vi "New Acquire.vi"() -> ()   [LabVIEW 2019]
uses:
  <vilib>/vision/NI_Vision_Development_Module.lvlib
panel:
  in  "Tab Control":T1(tab)
  out "Counts per Laser Shot :":dbl format="%#.1g"
  in  "Image Size (pixels) :":dbl=400.0
  in  "?":bool
  in  "Acquiring :":bool
  in  "Save?":bool
  in  "Mask Width (pixels) :":dbl
  in  "Mask Centre :":bool
  in  "Threshold Level (%) :":dbl
  in  "Image Centre (x,y) : 2":dbl=250.0
  in  "Image Centre (x,y) :":dbl=301.0
  in  "Symmetrise L/R :":bool
  in  "Symmetrise U/D :":bool
  in  "Centroiding :":bool
  out "Test View":dbl[][](graph)
  out "Integrated Signal Graph":dbl[](graph)
  out "Live Camera View":dbl[][](graph)
  out "PECD = LCP - RCP":dbl[][](graph)
  out "RCP":dbl[][](graph)
  out "LCP":dbl[][](graph)
  out "Elipticity :":dbl format="%#.2g"
  in  "RCP Position :":dbl=85.7
  in  "?":refnum<k7>(container)
  in  "?":refnum<k7>(container)
  out "of":dbl
  out "Scan :":dbl
  out "Progress :":u8(slide) scale=0.0..100.0
  out "of":dbl
  out "Shot :":dbl
  in  "Molecule :":string
  in  "OK Button 2":bool
  in  "No. of CPL Cycles :":dbl=1.0
  in  "Shots per Cycle :":dbl=100.0
  in  "HWP Zero Position :":dbl=3.9
  out "?":cluster{dbl[], dbl[]}(graph)
  out "PEELD = LEP - REP":dbl[][](graph)
  out "REP Image":dbl[][](graph)
  out "LEP Image":dbl[][](graph)
  out "?":dbl[](graph)
  in  "HWP Step Size :":dbl=2.5
  in  "LCP Position :":dbl=175.7
  in  "No. of Scans :":dbl=10.0
  out "Shot :":dbl
  out "of":dbl
  out "Elipticity : 2":dbl format="%#.2g"
  in  "RCP Position : 2":dbl=85.7
  in  "?":refnum<k7>(container)
  in  "?":refnum<k7>(container)
  out "of  3":dbl
  out "Scan : 2":dbl
  out "Progress : 2":u8(slide) scale=0.0..100.0
  out "of  3":dbl
  out "Shot : 3":dbl
  in  "Molecule : 2":string
  in  "OK Button 3":bool
  in  "No. of CPL Cycles : 2":dbl=1.0
  in  "Shots per Cycle : 2":dbl=100.0
  in  "HWP Zero Position : 2":dbl=3.9
  out "?":cluster{dbl[], dbl[]}(graph)
  out "PEELD = LEP - REP 2":dbl[][](graph)
  out "REP Image 2":dbl[][](graph)
  out "LEP Image 2":dbl[][](graph)
  out "?":dbl[](graph)
  in  "HWP Step Size : 2":dbl=2.5
  in  "LCP Position : 2":dbl=175.7
  in  "No. of Scans : 2":dbl=10.0
  out "Shot : 2":dbl
  out "of 2":dbl
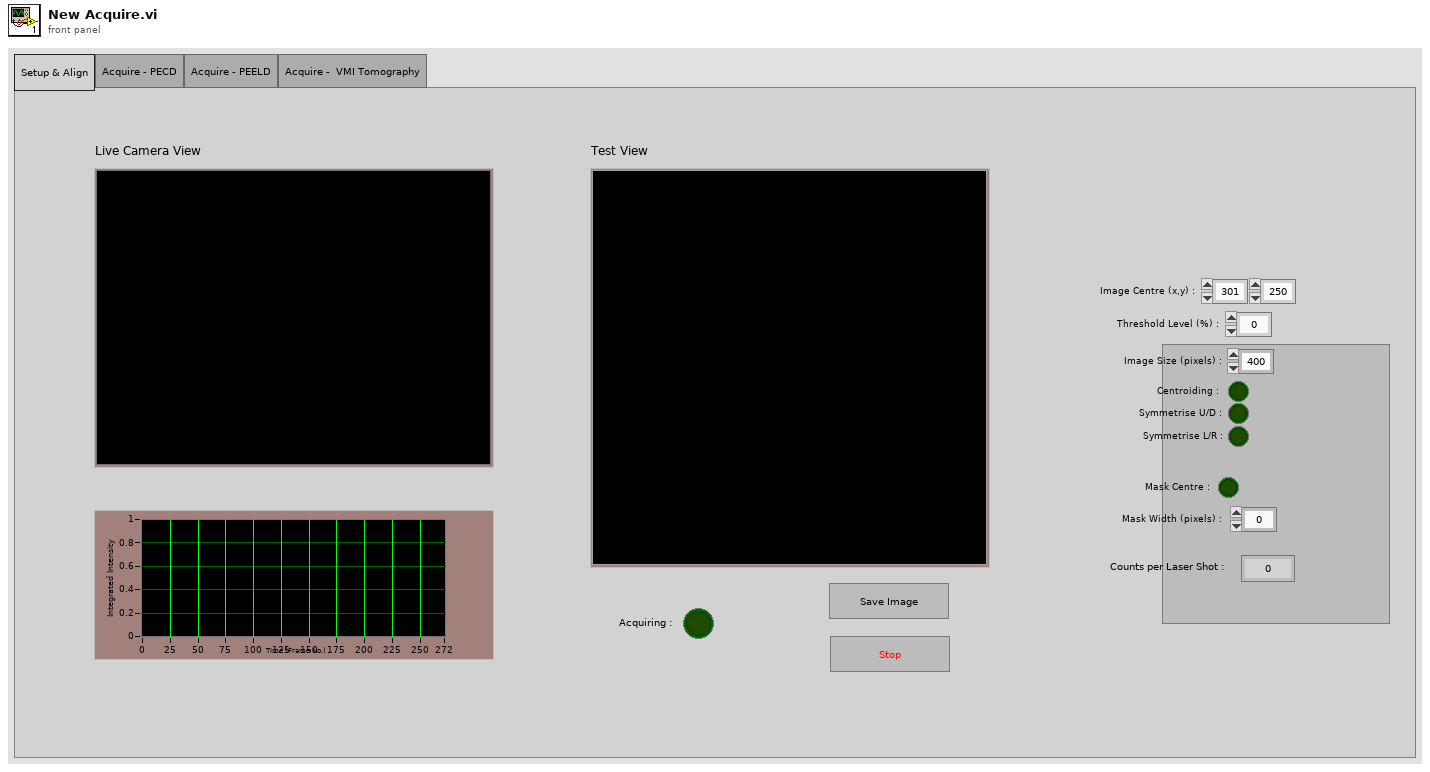
[diagram p1: front panel]
types:
  T1 = enum32{"Setup & Align", "Acquire - PECD", "Acquire - PEELD", "Acquire -  VMI Tomography"}
  T2 = typedef "Image Type" = u32
  T3 = typedef "IMAQ Image.ctl" = refnum<image>
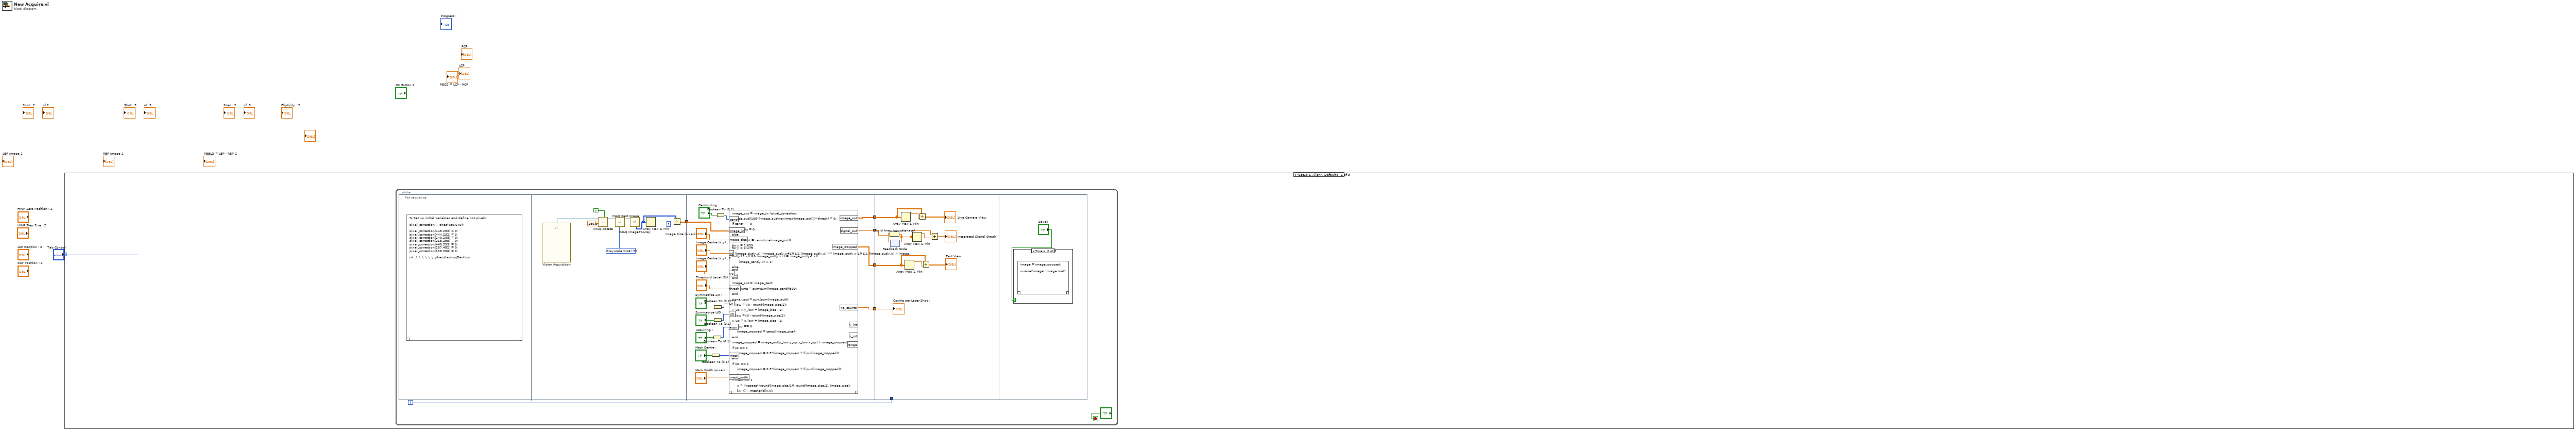
[diagram p0: block diagram]
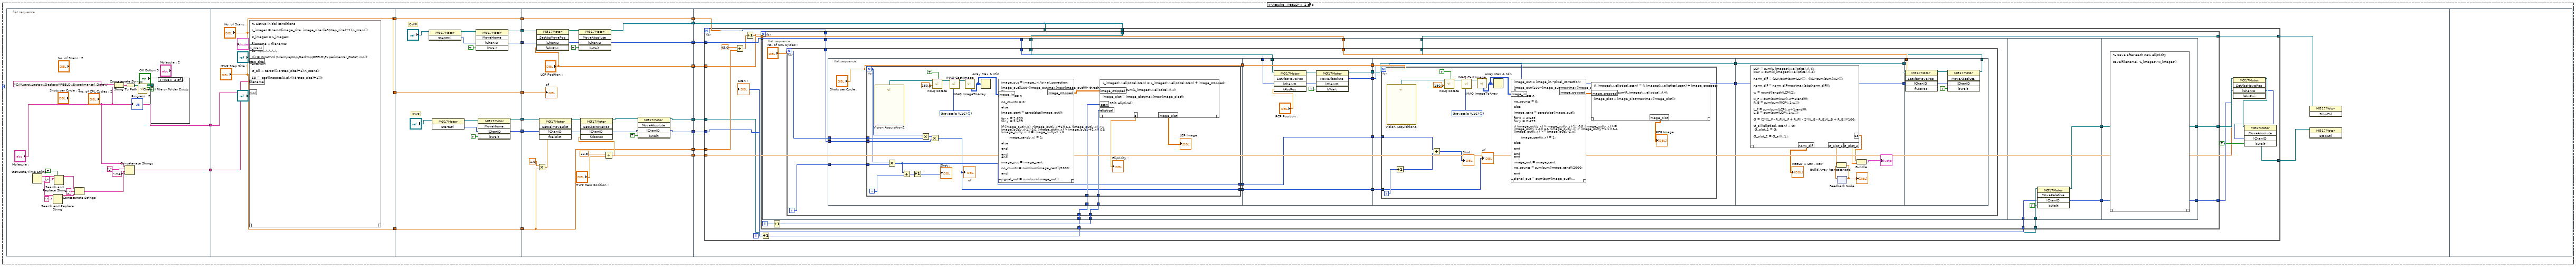
[diagram p3: hidden frame]
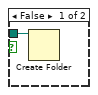
[diagram p4: hidden frame]
diagram:
  n1 = case shown="\"Setup & Align\", Default" "Tab Control" {
    frame "Setup & Align", Default {
      n2 = while {
        i -> [w4]
        stop <- "?" stop-if-true
        n3 = flat-sequence {
          tunnel: [w9] -> w8
          tunnel: w8 -> [w37]
          tunnel: [w36] -> w7
          tunnel: [w35] -> w5
          tunnel: [w31] -> w3
          tunnel: [w18] -> w2
          tunnel: w7 -> [w44]
          tunnel: w5 -> [w40]
          tunnel: w4 -> [_]
          tunnel: w3 -> [w41]
          tunnel: w2 -> [w38]
          frame #0 {
            n4 = script code="% Set up initial variables and define hot pixels\n\npixel_correction = ones(480,640);\n\npixel_correction(445,233) = 0;\npixel_correction(444,232) = 0\npixel_correction(240,208) = 0;\npixel_correction(268,295) = 0;\npixel_correction(440,333) = 0;\npixel_correction(257,482) = 0;\npixel_correction(128,286) = 0;\n\ncd ..\\..\\..\\..\\..\\..\\..\\Users\\Laptop\\Desktop"() -> ()  [unwired: 1 in, 1 out]
          }
          frame #1 {
            w17 = T2 7 items=["Grayscale (U8)", "Grayscale (I16)", "Grayscale (SGL)", "Complex (CSG)", "RGB (U32)", "HSL (U32)", "RGB (U64)", "Grayscale (U16)"] ("Image Type")
            n5 = call "Vision Acquisition"() -> ("Image Out"=w11:T3)  [unwired: 26 in, 1 out]
            n6 = call "IMAQ Rotate"("Maintain Size"=TRUE, "Angle (degrees)"=sgl 180.0, "Image Src"=w11) -> ("Image Dst Out"=w14:T3)  [unwired: 7 in, 1 out]
            n7 = call "IMAQ Cast Image"("Image Type"=w17, "Image Src"=w14) -> ("Image Dst Out"=w16:T3)  [unwired: 8 in, 1 out]
            n8 = call "IMAQ ImageToArray"("Image"=w16) -> ("Image Pixels (U16)"=w15:u16[][])  [unwired: 3 in, 4 out]
            n9 = Array Max & Min(array=w15) -> ()  [unwired: 4 out]
            n10 = Divide(x=w15, y=1) -> (x/y=w9:dbl[][])
          }
          frame #2 {
            n11 = Boolean To (0,1)(Boolean="Mask Centre :") -> (0, 1=w22:i16)
            n12 = Boolean To (0,1)(Boolean="Acquiring :") -> (0, 1=w25:i16)
            n13 = Boolean To (0,1)(Boolean="Symmetrise U/D :") -> (0, 1=w26:i16)
            n14 = Boolean To (0,1)(Boolean="Symmetrise L/R :") -> (0, 1=w29:i16)
            n15 = Boolean To (0,1)(Boolean="Centroiding :") -> (0, 1=w19:i16)
            n16 = script code="image_out = image_in.*pixel_correction;\n\nimage_out((100*(image_out/max(max(image_out))))<thresh) = 0;\n\nif centr == 0\n\nno_counts = 0;\n\nelse\n\nimage_cent = zeros(size(image_out));\n\nfor x = 2:639\nfor y = 2:479\n\nif (image_out(y,x) >image_out(y,x+1)) && (image_out(y,x) >= image_out(y,x-1)) && (image_out(y,x) > image_out(y+1,x)) && (image_out(y,x) >= image_out(y-1,x))\n\n       image_cent(y,x) = 1;\n\nelse\nend\n\nend\nend\n\nimage_out = image_cent;\n\nno_counts = sum(sum(image_cent))/500;\n\nend\n\nsignal_out = sum(sum(image_out));\n\ny_low = y0 - round(image_size/2);\n\ny_up = y_low + image_size - 1;\n\nx_low =x0 - round(image_size/2);\n\nx_up = x_low + image_size - 1;\n\nif acqu == 0\n\n     image_cropped = zeros(image_size);\n\nend\n\nimage_cropped = image_out(y_low:y_up,x_low:x_up) + image_cropped;\n\nif LR == 1\n\n     image_cropped = 0.5*(image_cropped + fliplr(image_cropped));\n\nend\n\nif UD == 1\n\n     image_cropped = 0.5*(image_cropped + flipud(image_cropped));\n\nend\n\nif mask == 1\n\n     x = linspace(-(round(image_size/2)), round(image_size/2), image_size);\n\n     [X, Y] = meshgrid(x,x);\n\n     R = sqrt(X.^2 + Y.^2);\n\n     mask_ = ones(size(R));\n\n     mask_(R<mask_width) = 0;\n\n     image_cropped = image_cropped.*mask_;\n\nend\n\nrange = 1:image_size;\n\ny_int = sum(image_cropped,1);\ny_int = y_int/max(y_int);\n\nx_int = sum(image_cropped,2);\nx_int = x_int/max(x_int);"("image_in"=w37, "image_size"="Image Size (pixels) :", "x0"="Image Centre (x,y) :", "y0"="Image Centre (x,y) : 2", "thresh"="Threshold Level (%) :", "LR"=w29, "UD"=w26, "acqu"=w25, "mask"=w22, "mask_width"="Mask Width (pixels) :", "centr"=w19) -> ("image_out"=w36:dbl[][], "signal_out"=w35:dbl, "image_cropped"=w31:dbl[][], "no_counts"=w18:dbl)  [unwired: 1 in, 4 out]
          }
          frame #3 {
            n17 = feedback #1() -> (w39:dbl[])  [unwired: 1 in]
            n18 = Build Array (concatenate)(w39, w40) -> (w48:dbl[])
            n19 = feedback-in #1(w48) -> ()
            n20 = Array Max & Min(array=w44) -> (max value=w45:dbl)  [unwired: 3 out]
            n21 = Array Max & Min(array=w41) -> (max value=w43:dbl)  [unwired: 3 out]
            n22 = Array Max & Min(array=w48) -> (max value=w47:dbl)  [unwired: 3 out]
            n23 = Divide(x=w44, y=w45) -> (x/y=→"Live Camera View":dbl[][])
            n24 = Divide(x=w41, y=w43) -> (x/y=→"Test View":dbl[][])
            n25 = Divide(x=w48, y=w47) -> (x/y=→"Integrated Signal Graph":dbl[])
            "Counts per Laser Shot :" <- w38
          }
          frame #4 {
            n26 = case shown="True" "Save?" {
              frame False {
              }
              frame True {
                n27 = script code="image = image_cropped;\n\nuisave('image','image.mat')"() -> ()  [unwired: 1 in, 1 out]
              }
            }
          }
        }
      }
    }
    frame "Acquire - PEELD" {
      n28 = flat-sequence {
        tunnel: [w72] -> w56
        tunnel: ["Molecule :"] -> w55
        tunnel: ["No. of Scans :"] -> w59
        tunnel: ["HWP Step Size :"] -> w57
        tunnel: w56 -> [w92]
        tunnel: w55 -> [w91]
        tunnel: ["No. of Scans :"] -> w53
        tunnel: [w100] -> w70
        tunnel: [w99] -> w69
        tunnel: [w98] -> w68
        tunnel: [w97] -> w67
        tunnel: [w96] -> w60
        tunnel: w59 -> [w96]
        tunnel: [w95] -> w58
        tunnel: w57 -> [w95]
        tunnel: w53 -> [w94]
        tunnel: [w94] -> w52
        tunnel: w70 -> [w133]
        tunnel: w69 -> [w132]
        tunnel: w68 -> [w131]
        tunnel: w67 -> [w130]
        tunnel: [w116] -> w66
        tunnel: [w122] -> w65
        tunnel: [w121] -> w64
        tunnel: ["LCP Position :"] -> w63
        tunnel: [w110] -> w62
        tunnel: [w119] -> w61
        tunnel: w60 -> [w119]
        tunnel: w58 -> [w110]
        tunnel: [w115] -> w54
        tunnel: w52 -> [w113]
        tunnel: [w112] -> w51
        tunnel: w66 -> [w143]
        tunnel: w65 -> [w139]
        tunnel: w64 -> [w141]
        tunnel: w63 -> [w140]
        tunnel: w62 -> [w136]
        tunnel: w61 -> [w135]
        tunnel: w54 -> [w142]
        tunnel: w51 -> [w134]
        frame #0 {
          n29 = Get Date/Time String() -> (date string=w83:string, time string=w80:string)  [unwired: 3 in]
          n30 = Search and Replace String(input string=w80, search string=":") -> (result string=w77:string)  [unwired: 6 in, 3 out]
          n31 = Search and Replace String(replace all?=TRUE ("replace all? (F)"), input string=w83, search string="/") -> (result string=w78:string)  [unwired: 5 in, 3 out]
          n32 = Concatenate Strings(w78, "_" ("string"), w77) -> (w74:string)
          n33 = Concatenate Strings("C:\\Users\\Laptop\\Desktop\\PEELD\\Experimental_Data\\", "Molecule :") -> (w84:string)
          n34 = Concatenate Strings("Molecule :", "_" ("string"), w74, ".mat" ("string")) -> (w72:string)
          n35 = String To Path(string=w84) -> (path=w87:path)
          n36 = call <vilib>:"Check if File or Folder Exists.vi"("path"=w87) -> ("file or folder exists?"=w86:bool, "dup path"=w85:path)  [unwired: 8 in, 1 out]
          n37 = case shown="True" w86 {
            tunnel: w85 -> [w89 _]
            frame False {
              n38 = Create Folder(path (use dialog)=w89) -> ()  [unwired: 2 in, 3 out]
            }
            frame True {
            }
          }
        }
        frame #1 {
          n39 = script code="% Set up initial conditions\n\nL_images = zeros([image_size, image_size,((45/step_size)+1),n_scans]);\n\nR_images = L_images;\n\nfilename = filename;\n\ncd  ..\\..\\..\\..\\..\\..\\\n\ndir = strcat('cd \\Users\\Laptop\\Desktop\\PEELD\\Experimental_Data\\',mol);\n\neval(dir)\n\nG_all = zeros(((45/step_size)+1),n_scans);\n\nS3 = -cos(linspace(0,pi,((45/step_size)+1)));"("n_scans"="No. of Scans :", "step_size"="HWP Step Size :", "filename"=w92, "mol"=w91) -> ()  [unwired: 1 in, 1 out]
        }
        frame #2 {
          # "HWP"
          # "QWP"
          n40 = invoke class="MG17Motor" method="StartCtrl"(reference="?") -> (reference out=w106:refnum<k7>, "StartCtrl"=w105:i32)  [unwired: 2 in, 1 out]
          n41 = invoke class="MG17Motor" method="StartCtrl"(reference="?") -> (reference out=w103:refnum<k7>, "StartCtrl"=w102:i32)  [unwired: 2 in, 1 out]
          n42 = invoke class="MG17Motor" method="MoveHome"(reference=w106, "lChanID"=w105, "bWait"=TRUE) -> (reference out=w100:refnum<k7>, "lChanID"=w98:i32)  [unwired: 2 in, 3 out]
          n43 = invoke class="MG17Motor" method="MoveHome"(reference=w103, "lChanID"=w102, "bWait"=TRUE) -> (reference out=w99:refnum<k7>, "lChanID"=w97:i32)  [unwired: 2 in, 3 out]
        }
        frame #3 {
          n44 = invoke class="MG17Motor" method="SetAbsMovePos"(reference=w133, "lChanID"=w131, "fAbsPos"="LCP Position :") -> (reference out=w129:refnum<k7>, "lChanID"=w128:i32)  [unwired: 2 in, 3 out]
          n45 = Multiply(x=-1.0, y=w110) -> (x*y=w111:dbl)
          n46 = invoke class="MG17Motor" method="SetRelMoveDist"(reference=w132, "lChanID"=w130, "fRelDist"=w111) -> (reference out=w126:refnum<k7>, "lChanID"=w125:i32)  [unwired: 2 in, 3 out]
          n47 = invoke class="MG17Motor" method="MoveAbsolute"(reference=w129, "lChanID"=w128, "bWait"=TRUE) -> (reference out=w122:refnum<k7>, "lChanID"=w121:i32)  [unwired: 2 in, 3 out]
          n48 = Add(x=22.5, y="HWP Zero Position :") -> (x+y=w112:dbl)
          n49 = invoke class="MG17Motor" method="SetAbsMovePos"(reference=w126, "lChanID"=w125, "fAbsPos"=w112) -> (reference out=w118:refnum<k7>, "lChanID"=w117:i32)  [unwired: 2 in, 3 out]
          n50 = invoke class="MG17Motor" method="MoveAbsolute"(reference=w118, "lChanID"=w117, "bWait"=TRUE) -> (reference out=w116:refnum<k7>, "lChanID"=w115:i32)  [unwired: 2 in, 3 out]
          "of" <- w113
        }
        frame #4 {
          n51 = for {
            N: w135 -> [w155]
            tunnel: w143 -> [w146]
            tunnel: w142 -> [w147]
            tunnel: w139 -> [_]
            tunnel: w141 -> [w162]
            tunnel: w140 -> [w161]
            tunnel: w139 -> [w163]
            tunnel: [w160] -> w138
            tunnel: [w159] -> w137
            tunnel: w136 -> [w157]
            tunnel: w134 -> [w148]
            i -> [w156]
            n52 = Divide(x=45.0, y=w157) -> (x/y=w144:dbl)
            n53 = Increment(x=w144) -> (x+1=w145:dbl)
            n54 = Increment(x=w156) -> (x+1=w154:i32)
            "Scan :" <- w154
            n55 = for {
              N: w145 -> [_]
              tunnel: w163 -> [w177]
              tunnel: w162 -> [w176]
              tunnel: w161 -> [w175]
              tunnel: w146 -> [w174]
              tunnel: w147 -> [w173]
              tunnel: [w172] -> w151
              tunnel: [w171] -> w150
              tunnel: [w170] -> w160
              tunnel: w154 -> [w167]
              tunnel: w155 -> [w164]
              i -> [w169]
              n56 = flat-sequence {
                tunnel: w177 -> [w184]
                tunnel: w176 -> [w183]
                tunnel: w175 -> [w182]
                tunnel: [w181] -> w170
                tunnel: w168 -> [w180]
                tunnel: w167 -> [w179]
                tunnel: w164 -> [w178]
                tunnel: w174 -> [w287]
                tunnel: w173 -> [w286]
                tunnel: [w285] -> w166
                tunnel: [w284] -> w165
                tunnel: [w288] -> w171
                tunnel: [w289] -> w172
                tunnel: w166 -> [w289]
                tunnel: w165 -> [w288]
                frame #0 {
                  n57 = for {
                    N: "No. of CPL Cycles :" -> [w191]
                    tunnel: w184 -> [w204]
                    tunnel: w183 -> [w203]
                    tunnel: w182 -> [w200]
                    tunnel: [w199] -> w181
                    tunnel: w180 -> [w198]
                    tunnel: w179 -> [w197]
                    tunnel: w178 -> [w190]
                    i -> [w192]
                    n58 = flat-sequence {
                      tunnel: ["Shots per Cycle :"] -> w206
                      tunnel: w198 -> [w213]
                      tunnel: w197 -> [w212]
                      tunnel: w192 -> [w211]
                      tunnel: w191 -> [w210]
                      tunnel: w190 -> [w209]
                      tunnel: [w208] -> w189
                      tunnel: [w207] -> w187
                      tunnel: w206 -> [w247]
                      tunnel: [w247] -> w205
                      tunnel: w204 -> [w243]
                      tunnel: w203 -> [w242]
                      tunnel: [w240] -> w202
                      tunnel: [w239] -> w201
                      tunnel: w189 -> [w238]
                      tunnel: [w238] -> w188
                      tunnel: w187 -> [w237]
                      tunnel: [w237] -> w186
                      tunnel: w205 -> [w252]
                      tunnel: [w251] -> w196
                      tunnel: w202 -> [w251]
                      tunnel: w201 -> [w250]
                      tunnel: [w250] -> w194
                      tunnel: w188 -> [w249]
                      tunnel: w186 -> [w248]
                      tunnel: w196 -> [w275]
                      tunnel: [w275] -> w195
                      tunnel: w194 -> [w274]
                      tunnel: [w274] -> w193
                      tunnel: w195 -> [w279]
                      tunnel: w193 -> [w278]
                      tunnel: w200 -> [w277]
                      tunnel: [w276] -> w199
                      frame #0 {
                        n59 = for {
                          N: "Shots per Cycle :" -> [w218]
                          tunnel: w213 -> [w228]
                          tunnel: w212 -> [w227]
                          tunnel: w211 -> [w225]
                          tunnel: w210 -> [w221]
                          tunnel: w209 -> [w219]
                          tunnel: [w217] -> w208
                          tunnel: [w216] -> w207
                          i -> [w224]
                          w236 = T2 7 items=["Grayscale (U8)", "Grayscale (I16)", "Grayscale (SGL)", "Complex (CSG)", "RGB (U32)", "HSL (U32)", "RGB (U64)", "Grayscale (U16)"] ("Image Type")
                          n60 = call "Vision Acquisition2"() -> ("Image Out"=w231:T3)  [unwired: 26 in, 1 out]
                          n61 = Multiply(x=w218, y=w225) -> (x*y=w217:i32)
                          n62 = Add(x=w217, y=w224) -> (x+y=w223:i32)
                          n63 = Increment(x=w223) -> (x+1=→"Shot :":i32)
                          n64 = Multiply(x=w218, y=w221) -> (x*y=w220:i32)
                          n65 = Multiply(x=w220, y=w219) -> (x*y=w216:i32)
                          "of" <- w216
                          n66 = call "IMAQ Rotate"("Maintain Size"=TRUE, "Angle (degrees)"=sgl 180.0, "Image Src"=w231) -> ("Image Dst Out"=w234:T3)  [unwired: 7 in, 1 out]
                          n67 = call "IMAQ Cast Image"("Image Type"=w236, "Image Src"=w234) -> ("Image Dst Out"=w235:T3)  [unwired: 8 in, 1 out]
                          n68 = call "IMAQ ImageToArray"("Image"=w235) -> ("Image Pixels (U16)"=w230:u16[][])  [unwired: 3 in, 4 out]
                          n69 = Array Max & Min(array=w230) -> ()  [unwired: 4 out]
                          n70 = script code="image_out = image_in.*pixel_correction;\n\nimage_out((100*(image_out/max(max(image_out))))<thresh) = 0;\n\nif centr == 0\n\nno_counts = 0;\n\nelse\n\nimage_cent = zeros(size(image_out));\n\nfor x = 2:639\nfor y = 2:479\n\nif (image_out(y,x) >image_out(y,x+1)) && (image_out(y,x) >= image_out(y,x-1)) && (image_out(y,x) > image_out(y+1,x)) && (image_out(y,x) >= image_out(y-1,x))\n\n       image_cent(y,x) = 1;\n\nelse\n\nend\n\nend\nend\n\nimage_out = image_cent;\n\nno_counts = sum(sum(image_cent))/2000;\n\nend\n\nsignal_out = sum(sum(image_out));\n\ny_low = y0 - round(image_size/2);\n\ny_up = y_low + image_size - 1;\n\nx_low =x0 - round(image_size/2);\n\nx_up = x_low + image_size - 1;\n\nimage_cropped = image_out(y_low:y_up,x_low:x_up);\n\nif LR == 1\n\n     image_cropped = 0.5*(image_cropped + fliplr(image_cropped));\n\nend\n\nif UD == 1\n\n     image_cropped = 0.5*(image_cropped + flipud(image_cropped));\n\nend\n\nif mask == 1\n\n     x = linspace(-(round(image_size/2)), round(image_size/2), image_size);\n\n     [X, Y] = meshgrid(x,x);\n\n     R = sqrt(X.^2 + Y.^2);\n\n     mask_ = ones(size(R));\n\n     mask_(R<mask_width) = 0;\n\n     image_cropped = image_cropped.*mask_;\n\nend\n\nrange = 1:image_size;\n\ny_int = sum(image_cropped,1);\ny_int = y_int/max(y_int);\n\nx_int = sum(image_cropped,2);\nx_int = x_int/max(x_int);"("image_in"=w230) -> ("image_cropped"=w229:dbl[][])  [unwired: 1 in, 1 out]
                          n71 = script code="L_images(:,:,eliptical,scan) = L_images(:,:,eliptical,scan) + image_cropped;\n\nimage_plot = sum(L_images(:,:,eliptical,:),4);\n\nimage_plot = image_plot/max(max(image_plot));\n\ne = S3(1,eliptical);"("image_cropped"=w229, "scan"=w227, "eliptical"=w228) -> ("image_plot"=→"LEP Image":dbl[][], "e"=→"Elipticity :":dbl)  [unwired: 1 in, 1 out]
                        }
                      }
                      frame #1 {
                        n72 = invoke class="MG17Motor" method="SetAbsMovePos"(reference=w243, "lChanID"=w242, "fAbsPos"="RCP Position :") -> (reference out=w246:refnum<k7>, "lChanID"=w245:i32)  [unwired: 2 in, 3 out]
                        n73 = invoke class="MG17Motor" method="MoveAbsolute"(reference=w246, "lChanID"=w245, "bWait"=TRUE) -> (reference out=w240:refnum<k7>, "MoveAbsolute"=w239:i32)  [unwired: 2 in, 3 out]
                      }
                      frame #2 {
                        n74 = for {
                          N: w252 -> [_]
                          tunnel: w249 -> [w257]
                          tunnel: w248 -> [w253]
                          i -> [w254]
                          w266 = T2 7 items=["Grayscale (U8)", "Grayscale (I16)", "Grayscale (SGL)", "Complex (CSG)", "RGB (U32)", "HSL (U32)", "RGB (U64)", "Grayscale (U16)"] ("Image Type")
                          n75 = call "Vision Acquisition3"() -> ("Image Out"=w261:T3)  [unwired: 26 in, 1 out]
                          n76 = Increment(x=w254) -> (x+1=w255:i32)
                          n77 = Add(x=w257, y=w255) -> (x+y=→"Shot :":i32)
                          n78 = call "IMAQ Rotate"("Maintain Size"=TRUE, "Angle (degrees)"=sgl 180.0, "Image Src"=w261) -> ("Image Dst Out"=w264:T3)  [unwired: 7 in, 1 out]
                          n79 = call "IMAQ Cast Image"("Image Type"=w266, "Image Src"=w264) -> ("Image Dst Out"=w265:T3)  [unwired: 8 in, 1 out]
                          n80 = call "IMAQ ImageToArray"("Image"=w265) -> ("Image Pixels (U16)"=w260:u16[][])  [unwired: 3 in, 4 out]
                          n81 = Array Max & Min(array=w260) -> ()  [unwired: 4 out]
                          n82 = script code="image_out = image_in.*pixel_correction;\n\nimage_out((100*(image_out/max(max(image_out))))<thresh) = 0;\n\nif centr == 0\n\nno_counts = 0;\n\nelse\n\nimage_cent = zeros(size(image_out));\n\nfor x = 2:639\nfor y = 2:479\n\nif (image_out(y,x) >image_out(y,x+1)) && (image_out(y,x) >= image_out(y,x-1)) && (image_out(y,x) > image_out(y+1,x)) && (image_out(y,x) >= image_out(y-1,x))\n\n       image_cent(y,x) = 1;\n\nelse\n\nend\n\nend\nend\n\nimage_out = image_cent;\n\nno_counts = sum(sum(image_cent))/2000;\n\nend\n\nsignal_out = sum(sum(image_out));\n\ny_low = y0 - round(image_size/2);\n\ny_up = y_low + image_size - 1;\n\nx_low =x0 - round(image_size/2);\n\nx_up = x_low + image_size - 1;\n\nimage_cropped = image_out(y_low:y_up,x_low:x_up);\n\nif LR == 1\n\n     image_cropped = 0.5*(image_cropped + fliplr(image_cropped));\n\nend\n\nif UD == 1\n\n     image_cropped = 0.5*(image_cropped + flipud(image_cropped));\n\nend\n\nif mask == 1\n\n     x = linspace(-(round(image_size/2)), round(image_size/2), image_size);\n\n     [X, Y] = meshgrid(x,x);\n\n     R = sqrt(X.^2 + Y.^2);\n\n     mask_ = ones(size(R));\n\n     mask_(R<mask_width) = 0;\n\n     image_cropped = image_cropped.*mask_;\n\nend\n\nrange = 1:image_size;\n\ny_int = sum(image_cropped,1);\ny_int = y_int/max(y_int);\n\nx_int = sum(image_cropped,2);\nx_int = x_int/max(x_int);"("image_in"=w260) -> ("image_cropped"=w259:dbl[][])  [unwired: 1 in, 1 out]
                          n83 = script code="R_images(:,:,eliptical,scan) = R_images(:,:,eliptical,scan) + image_cropped;\n\nimage_plot = sum(R_images(:,:,eliptical,:),4);\n\nimage_plot = image_plot/max(max(image_plot));"("image_cropped"=w259) -> ("image_plot"=→"REP Image":dbl[][])  [unwired: 1 in, 1 out]
                          "of" <- w253
                        }
                      }
                      frame #3 {
                        n84 = script code="LCP = sum(L_images(:,:,eliptical,:),4);\nRCP = sum(R_images(:,:,eliptical,:),4);\n\nnorm_dif = (LCP/sum(sum(LCP))) - (RCP/sum(sum(RCP)));\n\nnorm_dif = norm_dif/max(max(abs(norm_dif)));\n\nw = round(length(LCP)/2);\n\nR_F = sum(sum(RCP(:,w+1:end)));\nR_B = sum(sum(RCP(:,1:w)));\n\nL_F = sum(sum(LCP(:,w+1:end)));\nL_B = sum(sum(LCP(:,1:w)));\n\nG = (2*((L_F - R_F)/(L_F + R_F)) - 2*((L_B - R_B)/(L_B + R_B)))*100;\n\nG_all(eliptical, scan) = G;\n G_plot_1 = G;\n\nG_plot_2 = G_all(:,1);"() -> ("norm_dif"=→"PEELD = LEP - REP":dbl[][], "G_plot_1"=w272:dbl, "G_plot_2"=w268:dbl[], "S3"=w269:dbl[])  [unwired: 1 in, 1 out]
                        n85 = feedback #2() -> (w271:dbl[])  [unwired: 1 in]
                        n86 = Build Array (concatenate)(w272, w271) -> (w270:dbl[])
                        "?" <- w270
                        n87 = feedback-in #2(w270) -> ()
                        n88 = Bundle(w269, w268) -> (→"?":cluster{dbl[], dbl[]})  [unwired: 1 in]
                      }
                      frame #4 {
                        n89 = invoke class="MG17Motor" method="SetAbsMovePos"(reference=w279, "lChanID"=w278, "fAbsPos"=w277) -> (reference out=w282:refnum<k7>, "lChanID"=w281:i32)  [unwired: 2 in, 3 out]
                        n90 = invoke class="MG17Motor" method="MoveAbsolute"(reference=w282, "lChanID"=w281, "bWait"=TRUE) -> (reference out=w276:refnum<k7>)  [unwired: 2 in, 4 out]
                      }
                    }
                  }
                }
                frame #1 {
                  n91 = invoke class="MG17Motor" method="MoveRelative"(reference=w287, "lChanID"=w286, "bWait"=TRUE) -> (reference out=w285:refnum<k7>, "lChanID"=w284:i32)  [unwired: 2 in, 3 out]
                }
                frame #2 {
                  n92 = script code="% Save after each new elipticity\n\nsave(filename, 'L_images','R_images')"() -> ()  [unwired: 1 in, 1 out]
                }
              }
              n93 = Increment(x=w169) -> (x+1=w168:i32)
            }
            n94 = invoke class="MG17Motor" method="SetAbsMovePos"(reference=w151, "lChanID"=w150, "fAbsPos"=w148) -> (reference out=w153:refnum<k7>, "lChanID"=w152:i32)  [unwired: 2 in, 3 out]
            n95 = invoke class="MG17Motor" method="MoveAbsolute"(reference=w153, "lChanID"=w152, "bWait"=TRUE) -> (reference out=w159:refnum<k7>)  [unwired: 2 in, 4 out]
          }
          n96 = invoke class="MG17Motor" method="StopCtrl"(reference=w138) -> ()  [unwired: 2 in, 3 out]
          n97 = invoke class="MG17Motor" method="StopCtrl"(reference=w137) -> ()  [unwired: 2 in, 3 out]
        }
        frame #5 {
        }
      }
    }
    frame "Acquire - PECD" {
    }
  }
